vi "PH_SRDG645.get Hardware Information.vi"(0 "i ref in":refnum<vi>, 5 "error in":errorcluster) -> (14 "i ref out":refnum<vi>, 19 "error out":errorcluster)   [LabVIEW 2014, in "PH_SRDG645.lvlib"]
doc: "This VI queries hardware information as the serial number."
uses:
  PH_SRDG645.lvlib
  PH_Common/PH_Common.lvlib
  instr.lib/Stanford Research DG645/Stanford Research DG645 - Driver.lvlib
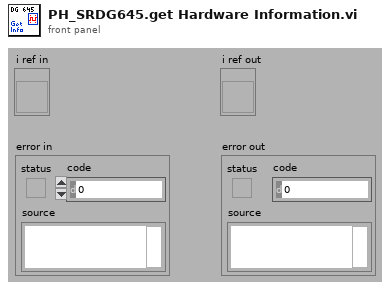
[diagram p1: front panel]
types:
  T1 = typedef "PH_SRDG645.lvlib/PH_SRDG645.i attribute.ctl" = cluster{"GUI Refs":cluster{"Delete":refnum<vi>, "Device Errors":refnum<vi>, "Trigger":refnum<vi>, "Default Name":refnum<vi>, "Firmware Revision":refnum<vi>, "Serial Number":refnum<vi>, "Model":refnum<vi>, "Visa resource name":refnum<vi>}, "Service ID Rate":i32, "Service IDs Channelinfo":i32[], "VISA resource name":refnum<visa-resource-name>, "Device Errors":cluster{"code":i32, "Text":string}[], "Trigger":T2, "Channels":cluster{"T1":T3, "A":T3, "B":T3, "C":T3, "D":T3, "E":T3, "F":T3, "G":T3, "H":T3}, "GUI Refs Channels":refnum<vi>[], "Outputs":cluster{"AB":cluster{"Level Offset [V]":dbl, "Amplitue [V]":dbl, "Polarity":i32}, "CD":cluster{"Level Offset [V]":dbl, "Amplitue [V]":dbl, "Polarity":i32}, "EF":cluster{"Level Offset [V]":dbl, "Amplitue [V]":dbl, "Polarity":i32}, "GH":cluster{"Level Offset [V]":dbl, "Amplitue [V]":dbl, "Polarity":i32}, "T0":cluster{"Level Offset [V]":dbl, "Amplitue [V]":dbl, "Polarity":i32}}, "GUI Refs Outputs":refnum<vi>[], "Serial Number":string, "Firmweare Revision":string, "Model":string}
  T2 = typedef "PH_SRDG645.lvlib/PH_SRDG645.Trigger.ctl" = cluster{"Source":i32, "Rate [Hz]":dbl, "Level [V]":dbl}
  T3 = typedef "PH_SRDG645.lvlib/PH_SRDG645.Channel Settings.ctl" = cluster{"Delay [s]":dbl, "relative to":i32}
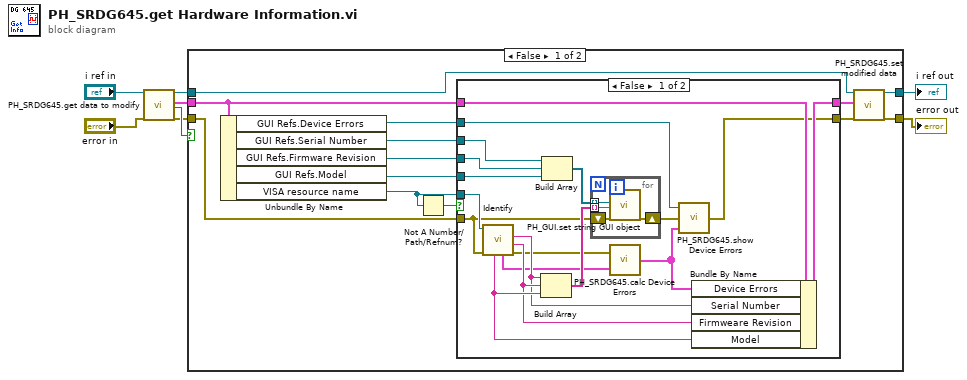
[diagram p0: block diagram]
diagram:
  n1 = call "PH_SRDG645.get data to modify.vi"("i ref in"="i ref in", "error in (no error)"="error in") -> ("i ref out"=w6:refnum<vi>, "i attribute"=w7:T1, "timed out"=w8:bool, "error out"=w1:errorcluster)  [unwired: 14 in]
  n2 = case shown="False" w8 {
    tunnel: w1 -> [w21 w46]
    tunnel: [w17 w47] -> w2
    tunnel: [w16 w46] -> w3
    tunnel: w6 -> [w9 w47]
    tunnel: w7 -> [w15 _]
    frame False {
      n3 = Unbundle By Name(w15) -> ("GUI Refs.Device Errors"=w12:refnum<vi>, "GUI Refs.Serial Number"=w20:refnum<vi>, "GUI Refs.Firmware Revision"=w19:refnum<vi>, "GUI Refs.Model"=w18:refnum<vi>, "VISA resource name"=w10:refnum<visa-resource-name>)
      n4 = Not A Number/Path/Refnum?(number/path/refnum=w10) -> (NaN/Path/Refnum?=w11:bool)
      n5 = case shown="False" w11 {
        tunnel: w21 -> [w24 w45]
        tunnel: w10 -> [w37 _]
        tunnel: w20 -> [w36 _]
        tunnel: w19 -> [w35 _]
        tunnel: w18 -> [w34 _]
        tunnel: w15 -> [w30 w44]
        tunnel: [w29 w44] -> w14
        tunnel: [w25 w45] -> w13
        tunnel: w12 -> [w26 _]
        frame False {
          n6 = call "Identify.vi"("error out"=w24, "VISA resource name"=w37) -> ("error out"=w27:errorcluster, "Instrument Firmware Revision"=w32:string, "Serial Number"=w31:string, "Device Errors"=w28:cluster{"code":i32, "Text":string}[], "Model"=w33:string)  [unwired: 2 in, 3 out]
          n7 = Build Array(w31, w32, w33) -> (w38:string[])
          n8 = Build Array(w36, w35, w34) -> (w39:refnum<vi>[])
          n9 = for {
            shift-right: [w43] -> w23
            shift-left: w24 -> [w42]
            tunnel: w39 -> [w41] mode=indexing
            tunnel: w38 -> [w40] mode=indexing
            n10 = call "PH_GUI.set string GUI object.vi"("GUI object Ref"=w41, "Text"=w40, "error in"=w42) -> ("error out"=w43:errorcluster)  [unwired: 16 in]
          }
          n11 = call "PH_SRDG645.calc Device Errors.vi"("Device Errors out"=w28, "SRDG 645 error out"=w27) -> ("calculate Device Errors"=w22:cluster{"code":i32, "Text":string}[])
          n12 = call "PH_SRDG645.show Device Errors.vi"("Device Errors"=w22, "error in"=w23, "Ref Device Errors"=w26) -> ("error out"=w25:errorcluster)
          n13 = Bundle By Name(cluster=w30, "Device Errors"=w22, "Serial Number"=w31, "Firmweare Revision"=w32, "Model"=w33) -> (w29:T1)
        }
        frame True {
        }
      }
      n14 = call "PH_SRDG645.set modified data.vi"("i ref in"=w9, "i attribute"=w14, "error in (no error)"=w13) -> ("i ref out"=w17:refnum<vi>, "error out"=w16:errorcluster)  [unwired: 15 in]
    }
    frame True {
    }
  }
  "error out" <- w3
  "i ref out" <- w2
